vi "TextToLines.vi"(6 "Remove Empty Lines?(T)":bool=TRUE, 8 "error in (no error)":errorcluster, 11 "string":string) -> (0 "error out":errorcluster, 3 "Lines":string[](array[string]))   [LabVIEW 2017, in "ini_configuration.lvlib"]
uses:
  ini_configuration.lvlib
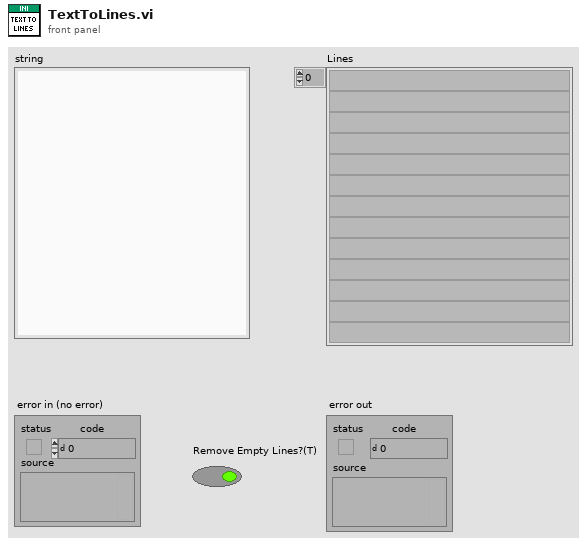
[diagram p1: front panel]
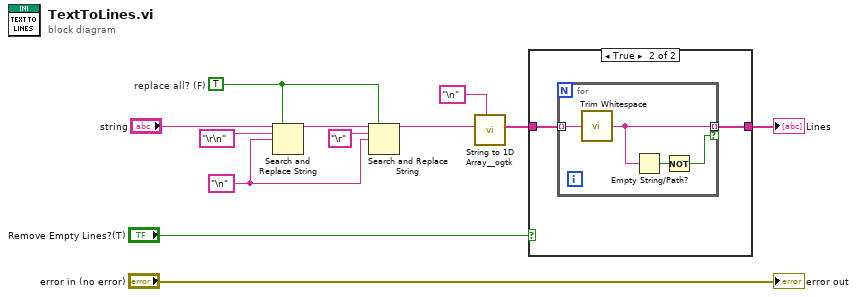
[diagram p0: block diagram]
diagram:
  w4 = TRUE  # replace all? (F)
  w5 = "\n" ("delimiter (Tab)")
  n1 = Search and Replace String(replace all?=w4, input string="string", search string="\r\n" ("delimiter (Tab)"), replace string=w5) -> (result string=w8:string)  [unwired: 4 in, 3 out]
  n2 = Search and Replace String(replace all?=w4, input string=w8, search string="\r" ("delimiter (Tab)"), replace string=w5) -> (result string=w6:string)  [unwired: 4 in, 3 out]
  n3 = call <userlib>:"String to 1D Array__ogtk.vi"("delimiter (Tab)"="\n", "string"=w6) -> ("Array of Strings"=w9:string[])  [unwired: 9 in]
  n4 = case shown="True" "Remove Empty Lines?(T)" {
    tunnel: [w13 w15] -> w11
    tunnel: w9 -> [w13 w14]
    frame False {
    }
    frame True {
      n5 = for {
        tunnel: w14 -> [w19] mode=indexing
        tunnel: [w18] -> w15 mode=indexing if=w16
        n6 = call <vilib>:"Trim Whitespace.vi"("string"=w19) -> ("trimmed string"=w18:string)  [unwired: 1 in]
        n7 = Empty String/Path?(string/path=w18) -> (empty?=w17:bool)
        n8 = Not(x=w17) -> (.not. x?=w16:bool)
      }
    }
  }
  "Lines" <- w11
  "error out" <- "error in (no error)"
